vi "ReadDynamixelPosition.vi"(8 "error in (no error)":errorcluster, 9 "VISA resource name":refnum<visa-resource-name>, 10 "DynamixelPositions Queue":refnum<queue>, 11 "Notifier References":T1) -> (0 "error out":errorcluster, 3 "Dynamixel positions":dbl[](array[numeric]))   [LabVIEW 2013]
doc: "Reads Dynamixel torque off of the indicated Dynamixel and writes it to a queue.\n\nEric Schneider, March 2014"
uses:
  Data/TypeDefs/Notifiers.ctl
  Data/TypeDefs/UTM Location.ctl
  Data/TypeDefs/Sail Set Suggestions.ctl
  Data/TypeDefs/Rudder Set Suggestions.ctl
  Data/TypeDefs/OverrideInformation.ctl
  Data/TypeDefs/OverrideMode.ctl
  Data/TypeDefs/MotorSetup.ctl
  Data/TypeDefs/DynamixelSetupInfo.ctl
  Data/TypeDefs/AirmarStatus.ctl
  Data/TypeDefs/HardwareOnline.ctl
  <instrlib>/Dynamixel Motor/Dynamixel Motor.lvlib
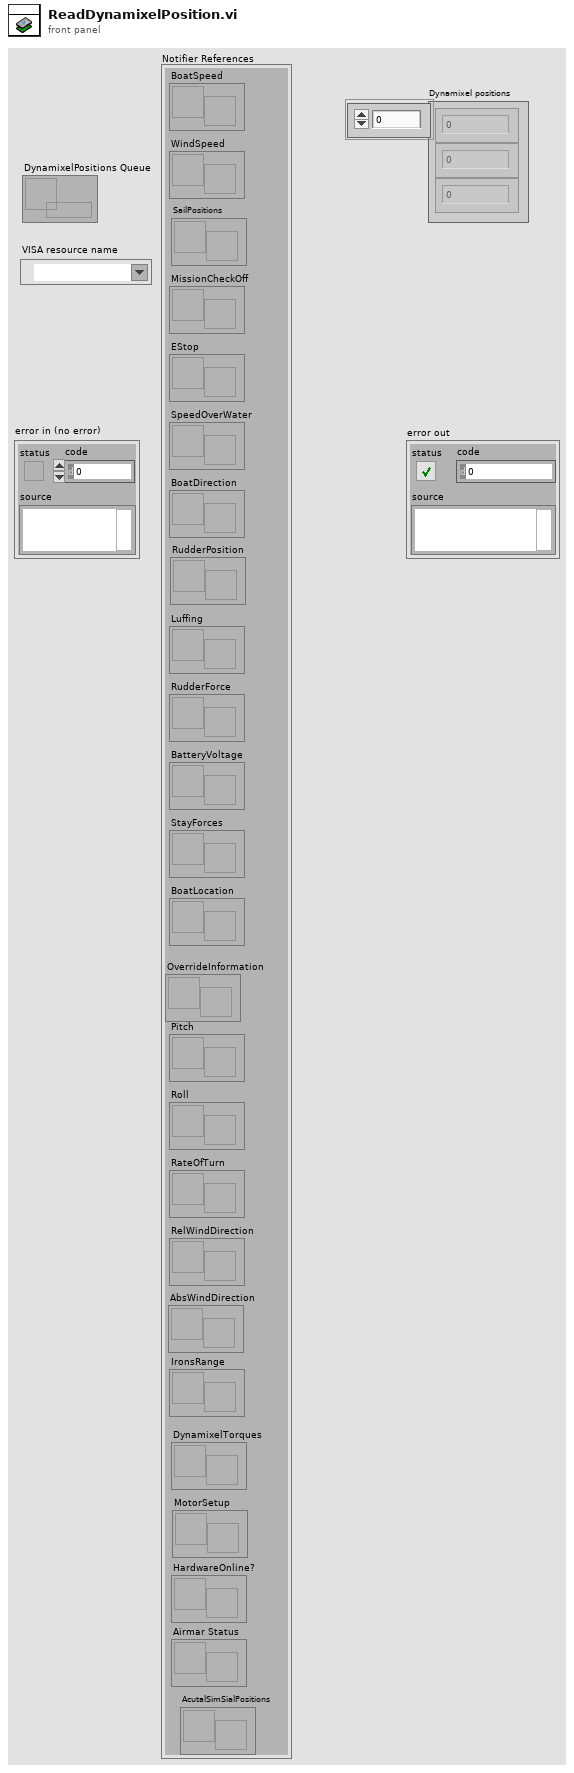
[diagram p1: front panel]
types:
  T1 = typedef "Notifiers.ctl" = cluster{"BoatSpeed":refnum<notifier>, "WindSpeed":refnum<notifier>, "MissionCheckOff":refnum<notifier>, "EStop":refnum<notifier>, "SpeedOverWater":refnum<notifier>, "BoatDirection":refnum<notifier>, "Luffing":refnum<notifier>, "RudderForce":refnum<notifier>, "BatteryVoltage":refnum<notifier>, "StayForces":refnum<notifier>, "BoatLocation":refnum<notifier>, "Pitch":refnum<notifier>, "Roll":refnum<notifier>, "RateOfTurn":refnum<notifier>, "RelWindDirection":refnum<notifier>, "SailPositions":refnum<notifier>, "RudderPosition":refnum<notifier>, "IronsRange":refnum<notifier>, "AbsWindDirection":refnum<notifier>, "OverrideInformation":refnum<notifier>, "DynamixelTorques":refnum<notifier>, "MotorSetup":refnum<notifier>, "Airmar Status":refnum<notifier>, "HardwareOnline?":refnum<notifier>, "AcutalSimSialPositions":refnum<notifier>}
  T2 = typedef "HardwareOnline.ctl" = cluster{"AirmarOnline":bool, "WindvaneOnline":bool, "HemisphereOnline":bool, "StayForceOnline":bool, "BatteryVoltageOnline":bool, "AccelerometerOnline":bool, "MainDynamixel Online":bool, "JibDynamixel Online":bool, "RudderDynamixel Online":bool}
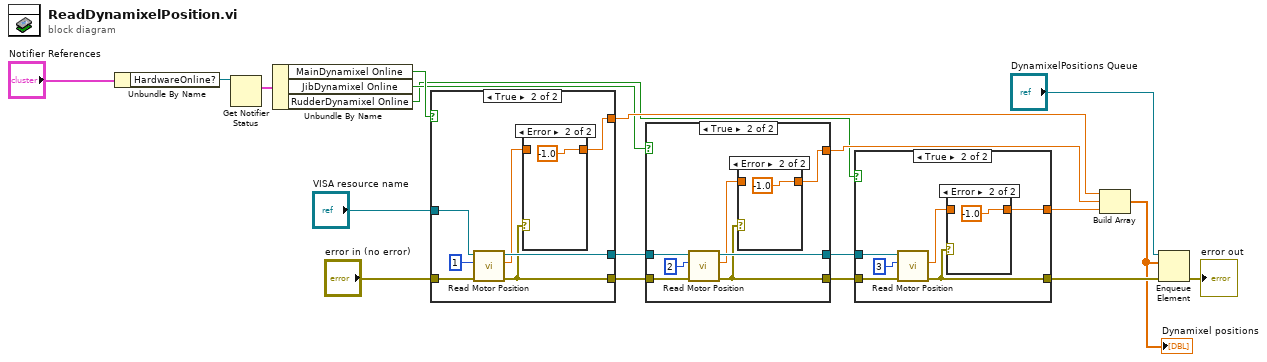
[diagram p0: block diagram]
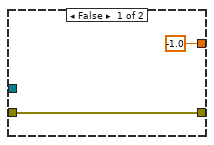
[diagram p2: hidden frame]
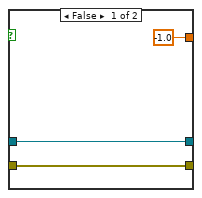
[diagram p4: hidden frame]
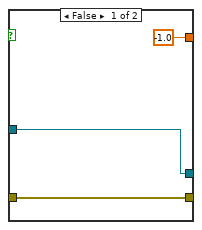
[diagram p6: hidden frame]
diagram:
  n1 = Unbundle By Name("Notifier References") -> ("HardwareOnline?"=w5:refnum<notifier>)
  n2 = Get Notifier Status(notifier=w5) -> (current notification=w4:T2)  [unwired: 1 in, 4 out]
  n3 = Unbundle By Name(w4) -> ("MainDynamixel Online"=w3:bool, "JibDynamixel Online"=w2:bool, "RudderDynamixel Online"=w1:bool)
  n4 = case shown="True" w3 {
    tunnel: "VISA resource name" -> [w21 w29]
    tunnel: "error in (no error)" -> [w20 w28]
    tunnel: [w21 w26] -> w16
    tunnel: [w20 w25] -> w15
    tunnel: [-1.0 ("Position (deg)") w23] -> w12
    frame False {
    }
    frame True {
      n5 = call <instrlib>:"Read Motor Position.vi"("error in (no error)"=w28, "Motor ID (0)"=u8 1, "VISA resource name"=w29) -> ("error out"=w25:errorcluster, "Position (deg)"=w24:dbl, "VISA resource name out"=w26:refnum<visa-resource-name>)  [unwired: 6 in]
      n6 = case shown="Error" w25 {
        tunnel: w24 -> [w30 _]
        tunnel: [w30 -1.0 ("Position (deg)")] -> w23
        frame No Error {
        }
        frame Error {
        }
      }
    }
  }
  n7 = case shown="True" w2 {
    tunnel: w16 -> [w32 w41]
    tunnel: w15 -> [w33 w40]
    tunnel: [w32 w39] -> w14
    tunnel: [w33 w37] -> w13
    tunnel: [-1.0 ("Position (deg)") w35] -> w11
    frame False {
    }
    frame True {
      n8 = call <instrlib>:"Read Motor Position.vi"("error in (no error)"=w40, "Motor ID (0)"=u8 2, "VISA resource name"=w41) -> ("error out"=w37:errorcluster, "Position (deg)"=w36:dbl, "VISA resource name out"=w39:refnum<visa-resource-name>)  [unwired: 6 in]
      n9 = case shown="Error" w37 {
        tunnel: w36 -> [w42 _]
        tunnel: [w42 -1.0 ("Position (deg)")] -> w35
        frame No Error {
        }
        frame Error {
        }
      }
    }
  }
  n10 = case shown="True" w1 {
    tunnel: w14 -> [_ w51]
    tunnel: w13 -> [w44 w50]
    tunnel: [-1.0 ("Position (deg)") w46] -> w10
    tunnel: [w44 w48] -> w9
    frame False {
    }
    frame True {
      n11 = call <instrlib>:"Read Motor Position.vi"("error in (no error)"=w50, "Motor ID (0)"=u8 3, "VISA resource name"=w51) -> ("error out"=w48:errorcluster, "Position (deg)"=w47:dbl)  [unwired: 6 in, 1 out]
      n12 = case shown="Error" w48 {
        tunnel: [w52 -1.0 ("Position (deg)")] -> w46
        tunnel: w47 -> [w52 _]
        frame No Error {
        }
        frame Error {
        }
      }
    }
  }
  n13 = Build Array(w12, w11, w10) -> (w7:dbl[])
  "Dynamixel positions" <- w7
  n14 = Enqueue Element(queue="DynamixelPositions Queue", element=w7, error in (no error)=w9) -> (error out=→"error out":errorcluster)  [unwired: 1 in, 2 out]
